vi "Ball HandlingBegin.vi"() -> ()   [LabVIEW 2019]
uses:
  <vilib>/Rock Robotics/SystemInterfaces/DIO/FPGA_DIOPWMChannel.ctl
  <vilib>/Rock Robotics/WPI/Solenoid/WPI_SolenoidChannel.ctl
  <vilib>/Rock Robotics/WPI/Solenoid/WPI_SolenoidValue.ctl
  <vilib>/Rock Robotics/WPI/SafetyOutput/WPI_SafetyOutputConfigMenu.ctl
  <vilib>/Rock Robotics/SystemInterfaces/DIO/FPGA_DIOChannel.ctl
  <vilib>/Rock Robotics/WPI/MotorControl/WPI_MotorControlOpen VictorSPX.vi
  <vilib>/Rock Robotics/WPI/MotorControl/WPI_MotorControlOpen SPARK.vi
  <vilib>/Rock Robotics/WPI/Solenoid/WPI_SolenoidOpenDouble.vi
  <vilib>/Rock Robotics/WPI/Solenoid/WPI_SolenoidSetEnum.vi
  <vilib>/Rock Robotics/WPI/Switch/WPI_SwitchOpenLimit.vi
panel:
  out "error out 2":errorcluster
  out "error out":errorcluster
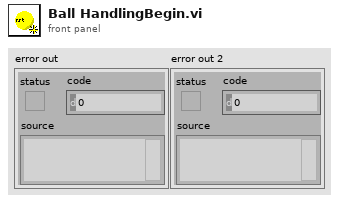
[diagram p1: front panel]
types:
  T1 = typedef "FPGA_DIOChannel.ctl" = enum8{"DIO 0", "DIO 1", "DIO 2", "DIO 3", "DIO 4", "DIO 5", "DIO 6", "DIO 7", "DIO 8", "DIO 9", "DIO MXP 0", "DIO MXP 1", "DIO MXP 2", "DIO MXP 3", "DIO MXP 4", "DIO MXP 5", "DIO MXP 6", "DIO MXP 7", "DIO MXP 8", "DIO MXP 9", "DIO MXP 10", "DIO MXP 11", "DIO MXP 12", "DIO MXP 13", "DIO MXP 14", "DIO MXP 15", "SPI Port CS1", "SPI Port CS2", "SPI Port CS3", "SPI Port MISO", "SPI Port MOSI", "Invalid"}
  T2 = typedef "WPI_SafetyOutputConfigMenu.ctl" = enum16{"Enable", "Disable"}
  T3 = typedef "WPI_SolenoidValue.ctl" = enum16{"Off", "On", "Forward", "Reverse"}
  T4 = typedef "WPI_SolenoidChannel.ctl" = enum8{"Solenoid 0", "Solenoid 1", "Solenoid 2", "Solenoid 3", "Solenoid 4", "Solenoid 5", "Solenoid 6", "Solenoid 7", "Invalid"}
  T5 = typedef "FPGA_DIOPWMChannel.ctl" = enum8{"PWM 0", "PWM 1", "PWM 2", "PWM 3", "PWM 4", "PWM 5", "PWM 6", "PWM 7", "PWM 8", "PWM 9", "PWM MXP 0", "PWM MXP 1", "PWM MXP 2", "PWM MXP 3", "PWM MXP 4", "PWM MXP 5", "PWM MXP 6", "PWM MXP 7", "PWM MXP 8", "PWM MXP 9", "Invalid"}
  T6 = typedef "WPI_SwitchDevRef.ctl" = cluster{"DevStatus":errorcluster, "DIO Channel":T1, "CntIndex":T7, "Normally Closed":bool}
  T7 = typedef "FPGA_CounterCtrSystemIndex.ctl" = enum8{"Ctr 0", "Ctr 1", "Ctr 2", "Ctr 3", "Ctr 4", "Ctr 5", "Ctr 6", "Ctr 7", "Invalid"}
  T8 = typedef "WPI_MotorControlDeviceRef.ctl" = cluster{"DeviceStatus":errorcluster, "Type":T9, "PWM":cluster{"PWM Channel":T5, "DeadBand":T10}, "CAN":cluster{"Device Number":u8, "SetOutput VI Ref":variant, "GetOutput VI Ref":variant, "Enable VI Ref":variant, "Disable VI Ref":variant, "Data":variant}, "Invert":bool, "DIO PWM":cluster{"PWM \"Enable\" Channel":T5, "DIOChannel":T1, "PWM Rate":dbl}}
  T9 = typedef "WPI_MotorControlType.ctl" = enum16{"PWM", "CAN", "DIO PWM"}
  T10 = typedef "WPI_PWMDeadband.ctl" = cluster{"Name":string, "maxPositivePwm":i32, "minPositivePwm":i32, "centerPwm":i32, "maxNegativePwm":i32, "minNegativePwm":i32, "angularRange":u16}
  T11 = typedef "WPI_SolenoidDevRef.ctl" = cluster{"DevStatus":errorcluster, "Pneumatics Control Module":u8, "Forward Solenoid Channel":T4, "Reverse Solenoid Channel":T4}
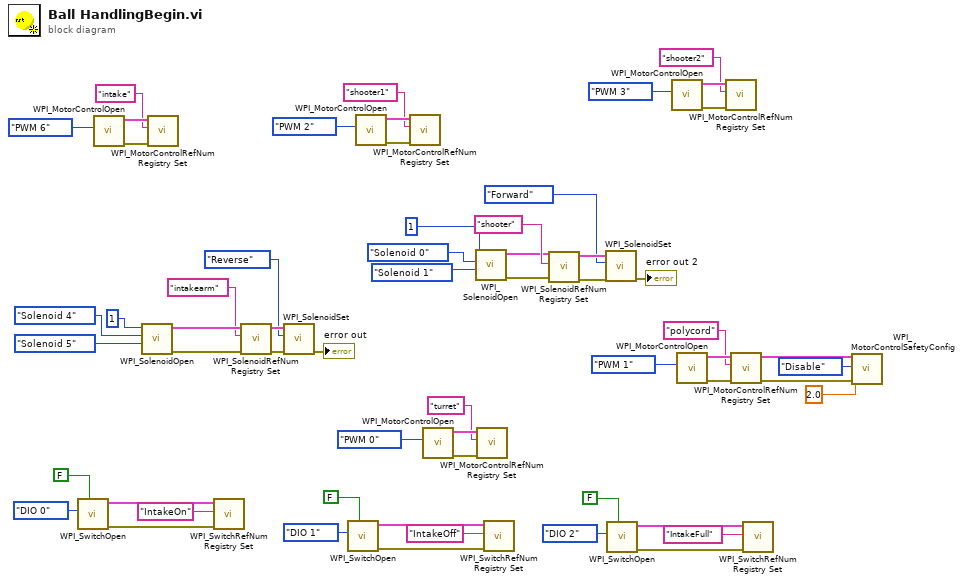
[diagram p0: block diagram]
diagram:
  n1 = call-poly <vilib>:"WPI_SwitchOpen.vi"("Normally Closed"=FALSE, "DIO Channel"=FPGA_DIOChannel."DIO 0") -> ("error out"=w14:errorcluster, "SwitchDevRef"=w13:T6)  [unwired: 8 in]
  n2 = call-poly <vilib>:"WPI_MotorControlOpen.vi"("PWM Channel"=FPGA_DIOPWMChannel."PWM 6") -> ("error out"=w58:errorcluster, "MotorControlDeviceRef"=w57:T8)  [unwired: 9 in]
  n3 = call-poly <vilib>:"WPI_SolenoidOpen.vi"("Reverse Solenoid Channel"=WPI_SolenoidChannel."Solenoid 5", "Forward Solenoid Channel"=WPI_SolenoidChannel."Solenoid 4" ("Solenoid Channel"), "Pneumatics Control Module (0)"=u8 1) -> ("error out"=w27:errorcluster, "SolenoidDevRef"=w26:T11)  [unwired: 7 in]
  n4 = call <vilib>:"WPI_MotorControlRefNum Registry Set.vi"("error in (no error)"=w58, "refnum name"="intake", "MotorControlDevRef"=w57) -> ()  [unwired: 7 in, 2 out]
  n5 = call <vilib>:"WPI_SwitchRefNum Registry Set.vi"("error in (no error)"=w14, "refnum name"="IntakeOn", "SwitchDevRef"=w13) -> ()  [unwired: 7 in, 2 out]
  n6 = call <vilib>:"WPI_SolenoidRefNum Registry Set.vi"("error in (no error)"=w27, "refnum name"="intakearm", "SolenoidDevRef"=w26) -> ("error out"=w24:errorcluster, "SolenoidDevRef"=w23:T11)  [unwired: 7 in]
  n7 = call-poly <vilib>:"WPI_SolenoidSet.vi"("error in (no error)"=w24, "Value"=WPI_SolenoidValue."Reverse", "SolenoidDevRef"=w23) -> ("error out"=→"error out":errorcluster)  [unwired: 7 in, 1 out]
  n8 = call-poly <vilib>:"WPI_SwitchOpen.vi"("Normally Closed"=FALSE, "DIO Channel"=FPGA_DIOChannel."DIO 1") -> ("error out"=w9:errorcluster, "SwitchDevRef"=w10:T6)  [unwired: 8 in]
  n9 = call-poly <vilib>:"WPI_MotorControlOpen.vi"("PWM Channel"=FPGA_DIOPWMChannel."PWM 2") -> ("error out"=w55:errorcluster, "MotorControlDeviceRef"=w54:T8)  [unwired: 9 in]
  n10 = call <vilib>:"WPI_MotorControlRefNum Registry Set.vi"("error in (no error)"=w55, "refnum name"="shooter1", "MotorControlDevRef"=w54) -> ()  [unwired: 7 in, 2 out]
  n11 = call-poly <vilib>:"WPI_MotorControlOpen.vi"("PWM Channel"=FPGA_DIOPWMChannel."PWM 0") -> ("error out"=w37:errorcluster, "MotorControlDeviceRef"=w36:T8)  [unwired: 9 in]
  n12 = call-poly <vilib>:"WPI_SolenoidOpen.vi"("Reverse Solenoid Channel"=WPI_SolenoidChannel."Solenoid 1", "Forward Solenoid Channel"=WPI_SolenoidChannel."Solenoid 0" ("Solenoid Channel"), "Pneumatics Control Module (0)"=u8 1) -> ("error out"=w41:errorcluster, "SolenoidDevRef"=w40:T11)  [unwired: 7 in]
  n13 = call <vilib>:"WPI_MotorControlRefNum Registry Set.vi"("error in (no error)"=w37, "refnum name"="turret", "MotorControlDevRef"=w36) -> ()  [unwired: 7 in, 2 out]
  n14 = call <vilib>:"WPI_SwitchRefNum Registry Set.vi"("error in (no error)"=w9, "refnum name"="IntakeOff", "SwitchDevRef"=w10) -> ()  [unwired: 7 in, 2 out]
  n15 = call <vilib>:"WPI_SolenoidRefNum Registry Set.vi"("error in (no error)"=w41, "refnum name"="shooter", "SolenoidDevRef"=w40) -> ("error out"=w45:errorcluster, "SolenoidDevRef"=w44:T11)  [unwired: 7 in]
  n16 = call-poly <vilib>:"WPI_SolenoidSet.vi"("error in (no error)"=w45, "Value"=WPI_SolenoidValue."Forward", "SolenoidDevRef"=w44) -> ("error out"=→"error out 2":errorcluster)  [unwired: 7 in, 1 out]
  n17 = call-poly <vilib>:"WPI_SwitchOpen.vi"("Normally Closed"=FALSE, "DIO Channel"=FPGA_DIOChannel."DIO 2") -> ("error out"=w4:errorcluster, "SwitchDevRef"=w3:T6)  [unwired: 8 in]
  n18 = call-poly <vilib>:"WPI_MotorControlOpen.vi"("PWM Channel"=FPGA_DIOPWMChannel."PWM 3") -> ("error out"=w52:errorcluster, "MotorControlDeviceRef"=w51:T8)  [unwired: 9 in]
  n19 = call-poly <vilib>:"WPI_MotorControlOpen.vi"("PWM Channel"=FPGA_DIOPWMChannel."PWM 1") -> ("error out"=w48:errorcluster, "MotorControlDeviceRef"=w47:T8)  [unwired: 9 in]
  n20 = call <vilib>:"WPI_MotorControlRefNum Registry Set.vi"("error in (no error)"=w52, "refnum name"="shooter2", "MotorControlDevRef"=w51) -> ()  [unwired: 7 in, 2 out]
  n21 = call <vilib>:"WPI_MotorControlRefNum Registry Set.vi"("error in (no error)"=w48, "refnum name"="polycord", "MotorControlDevRef"=w47) -> ("error out"=w20:errorcluster, "MotorControlDevRef"=w19:T8)  [unwired: 7 in]
  n22 = call <vilib>:"WPI_SwitchRefNum Registry Set.vi"("error in (no error)"=w4, "refnum name"="IntakeFull", "SwitchDevRef"=w3) -> ()  [unwired: 7 in, 2 out]
  n23 = call <vilib>:"WPI_MotorControlSafetyConfig.vi"("error in (no error)"=w20, "timeout (s)"=2.0, "mode"=WPI_SafetyOutputConfigMenu."Disable", "MotorControlDevRef"=w19) -> ()  [unwired: 6 in, 2 out]
